vi "Close Notifiers.vi"(8 "error in":errorcluster, 11 "Notifiers":T1) -> (0 "error out":errorcluster)   [LabVIEW 2014]
uses:
  Notifiers.ctl
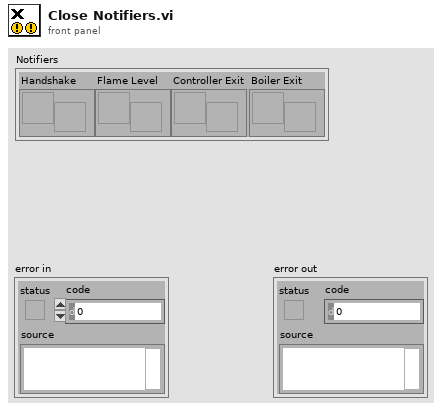
[diagram p1: front panel]
types:
  T1 = typedef "Notifiers.ctl" = cluster{"Handshake":refnum<notifier>, "Flame Level":refnum<notifier>, "Controller Exit":refnum<notifier>, "Boiler Exit":refnum<notifier>}
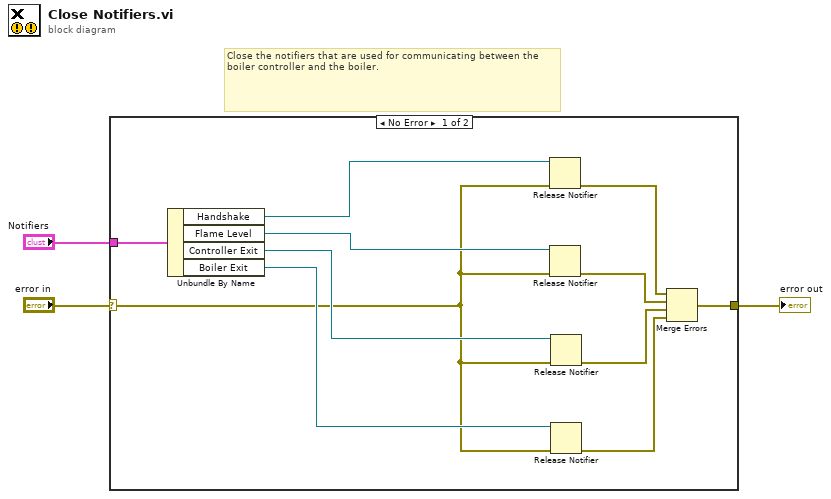
[diagram p0: block diagram]
diagram:
  # "Close the notifiers that are used for communicating between the boiler controller and the boiler."
  n1 = case shown="No Error" "error in" {
    selector: "error in" -> [w7 w15]
    tunnel: "Notifiers" -> [w14 _]
    tunnel: [w13 w15] -> w1
    frame No Error {
      n2 = Unbundle By Name(w14) -> ("Handshake"=w8:refnum<notifier>, "Flame Level"=w9:refnum<notifier>, "Controller Exit"=w10:refnum<notifier>, "Boiler Exit"=w12:refnum<notifier>)
      n3 = Release Notifier(notifier=w8, error in (no error)=w7) -> (error out=w4:errorcluster)  [unwired: 1 in, 2 out]
      n4 = Release Notifier(notifier=w9, error in (no error)=w7) -> (error out=w5:errorcluster)  [unwired: 1 in, 2 out]
      n5 = Release Notifier(notifier=w10, error in (no error)=w7) -> (error out=w6:errorcluster)  [unwired: 1 in, 2 out]
      n6 = Release Notifier(notifier=w12, error in (no error)=w7) -> (error out=w11:errorcluster)  [unwired: 1 in, 2 out]
      n7 = Merge Errors(w4, w5, w6, w11) -> (w13:errorcluster)
    }
    frame Error {
    }
  }
  "error out" <- w1
